vi "ADC_sparkle_remove.vi"(11 "Input Waveform":i64[](graph)) -> (3 "Output Waveform":dbl[](graph))   [LabVIEW 2016]
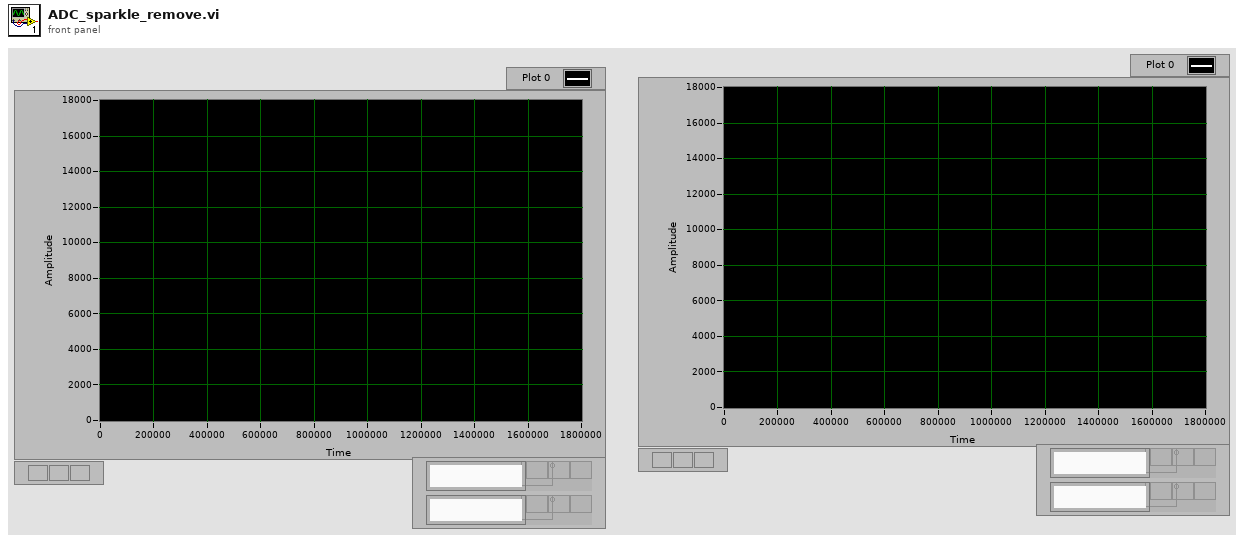
[diagram p1: front panel]
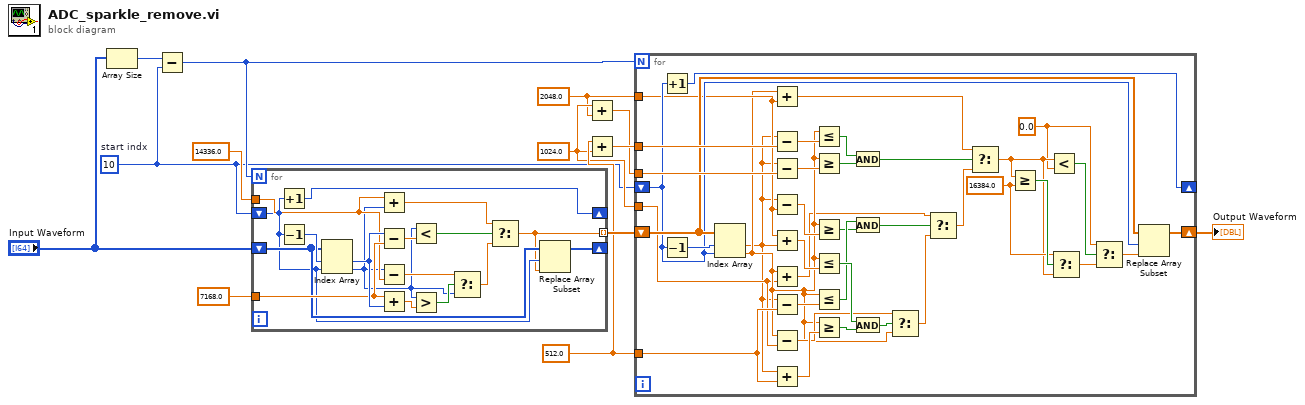
[diagram p0: block diagram]
diagram:
  w8 = 1024.0 ("disabled index (col)")
  w7 = 2048.0 ("disabled index (col)")
  w10 = 512.0 ("disabled index (col)")
  w3 = 10  # start indx
  n1 = Array Size(array="Input Waveform") -> (size(s)=w5:i32)
  n2 = Subtract(x=w5, y=w3) -> (x-y=w4:i32)
  n3 = for {
    N: w4 -> [_]
    shift-right: [w27] -> _
    shift-left: w3 -> [w15]
    tunnel: 7168.0 ("disabled index (col)") -> [w25]
    tunnel: 14336.0 ("disabled index (col)") -> [w23]
    tunnel: [w14] -> w11 mode=indexing
    shift-right: [w17] -> _
    shift-left: "Input Waveform" -> [w16]
    n4 = Increment(x=w15) -> (x+1=w27:i32)
    n5 = Decrement(x=w15) -> (x-1=w18:i32)
    n6 = Index Array(array=w16, index #1=w18, index #2=w15) -> (element #1=w26:i64, element #2=w20:i64)
    n7 = Add(x=w23, y=w20) -> (x+y=w22:dbl)
    n8 = Subtract(x=w26, y=w25) -> (x-y=w24:dbl)
    n9 = Subtract(x=w20, y=w23) -> (x-y=w28:dbl)
    n10 = Add(x=w25, y=w26) -> (x+y=w30:dbl)
    n11 = Less?(x=w20, y=w24) -> (x < y?=w21:bool)
    n12 = Greater?(x=w20, y=w30) -> (0:w29:bool)
    n13 = Select(t=w28, s=w29, f=w20) -> (s? t:f=w19:dbl)
    n14 = Select(t=w22, s=w21, f=w19) -> (s? t:f=w14:dbl)
    n15 = Replace Array Subset(array=w16, new element=w14, index=w15) -> (w17:i64[])
  }
  n16 = Add(x=w8, y=w7) -> (x+y=w6:dbl)
  n17 = Add(x=w10, y=w8) -> (x+y=w9:dbl)
  n18 = for {
    N: w4 -> [_]
    shift-right: [w54] -> w1
    shift-left: w11 -> [w55]
    shift-right: [w53] -> _
    shift-left: w3 -> [w52]
    tunnel: w10 -> [w51]
    tunnel: w7 -> [w47]
    tunnel: w8 -> [w43]
    tunnel: w9 -> [w61]
    tunnel: w6 -> [w59]
    w33 = 0.0 ("disabled index (col)")
    w36 = 16384.0 ("disabled index (col)")
    n19 = Increment(x=w52) -> (x+1=w53:i32)
    n20 = Decrement(x=w52) -> (x-1=w69:i32)
    n21 = Index Array(array=w55, index #1=w69, index #2=w52) -> (element #1=w42:dbl, element #2=w44:dbl)
    n22 = Add(x=w44, y=w47) -> (x+y=w40:dbl)
    n23 = Subtract(x=w42, y=w61) -> (x-y=w62:dbl)
    n24 = Subtract(x=w42, y=w59) -> (x-y=w60:dbl)
    n25 = Subtract(x=w42, y=w47) -> (x-y=w48:dbl)
    n26 = Add(x=w47, y=w42) -> (x+y=w67:dbl)
    n27 = Add(x=w44, y=w43) -> (x+y=w41:dbl)
    n28 = Subtract(x=w42, y=w51) -> (x-y=w50:dbl)
    n29 = Subtract(x=w44, y=w43) -> (x-y=w63:dbl)
    n30 = Add(x=w42, y=w51) -> (x+y=w68:dbl)
    n31 = Less Or Equal?(x=w44, y=w62) -> (x <= y?=w57:bool)
    n32 = Greater Or Equal?(x=w44, y=w60) -> (x >= y?=w58:bool)
    n33 = Greater Or Equal?(x=w44, y=w48) -> (x >= y?=w46:bool)
    n34 = Less Or Equal?(x=w44, y=w67) -> (x <= y?=w65:bool)
    n35 = Less Or Equal?(x=w44, y=w50) -> (x <= y?=w49:bool)
    n36 = Greater Or Equal?(x=w44, y=w68) -> (x >= y?=w66:bool)
    n37 = And(x=w57, y=w58) -> (x .and. y?=w39:bool)
    n38 = And(x=w49, y=w46) -> (x .and. y?=w38:bool)
    n39 = And(x=w65, y=w66) -> (x .and. y?=w64:bool)
    n40 = Select(t=w63, s=w64, f=w44) -> (s? t:f=w56:dbl)
    n41 = Select(t=w41, s=w38, f=w56) -> (s? t:f=w45:dbl)
    n42 = Select(t=w40, s=w39, f=w45) -> (s? t:f=w35:dbl)
    n43 = Greater Or Equal?(x=w35, y=w36) -> (x >= y?=w37:bool)
    n44 = Less?(x=w35, y=w33) -> (x < y?=w34:bool)
    n45 = Select(t=w36, s=w37, f=w35) -> (s? t:f=w32:dbl)
    n46 = Select(t=w33, s=w34, f=w32) -> (s? t:f=w31:dbl)
    n47 = Replace Array Subset(array=w55, new element=w31, index=w52) -> (w54:dbl[])
  }
  "Output Waveform" <- w1
